vi "Number to Formatted String.vi"(6 "In 2":dbl, 7 "In 1":dbl) -> (2 "Out":string)   [LabVIEW 2012]
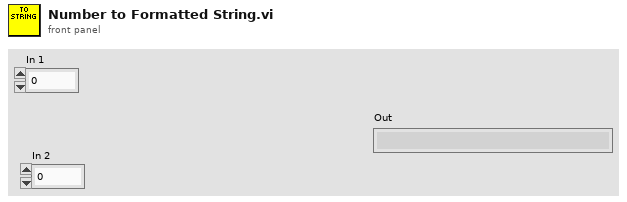
[diagram p1: front panel]
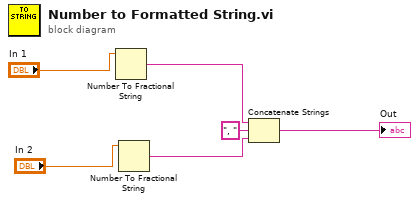
[diagram p0: block diagram]
diagram:
  n1 = Number To Fractional String(number="In 1") -> (F-format string=w4:string)  [unwired: 3 in]
  n2 = Number To Fractional String(number="In 2") -> (F-format string=w2:string)  [unwired: 3 in]
  n3 = Concatenate Strings(w4, ", " ("string"), w2) -> (→"Out":string)
